vi "InitBB.vi"(8 "Error In":errorcluster, 9 "ID":string, 10 "Active":bool, 11 "BB-Series in":refnum<class "BB-Series.lvclass">) -> (0 "Error Out":errorcluster, 3 "BB-Series out":refnum<class "BB-Series.lvclass">)   [LabVIEW 2021, in "BB-Series.lvclass"]
uses:
  BB-Series.lvclass
  BB-Series.lvclass/BB-Series.ctl
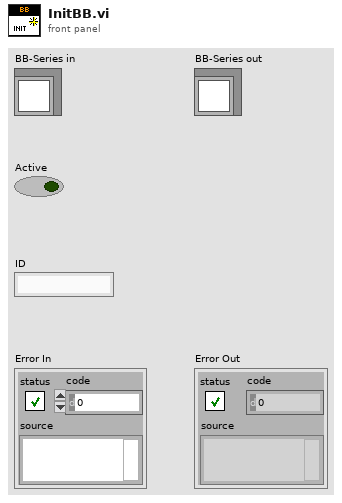
[diagram p1: front panel]
types:
  T1 = enum16{"Q-Series", "BB-Series", "C-Series", "R-Series"}
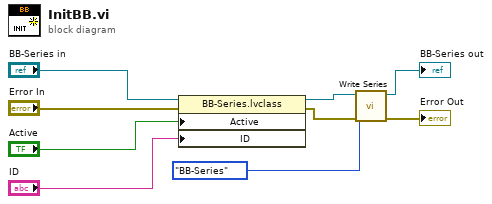
[diagram p0: block diagram]
diagram:
  n1 = property class="BB-Series.lvclass"(reference="BB-Series in", error in="Error In", "Active"="Active", "ID"="ID") -> (reference out=w5:refnum<class "BB-Series.lvclass">, error out=w4:errorcluster)
  n2 = call-dynamic "Write Series.vi"("error in (no error)"=w4, "Series"=T1."BB-Series", "Astromech droid in"=w5) -> ("error out"=→"Error Out":errorcluster, "Astromech droid out"=→"BB-Series out":refnum<class "BB-Series.lvclass">)  [unwired: 7 in]
